vi "Robot Global Data.vi"() -> ()   [LabVIEW 2014]
doc: "This global VI can contain as many global variables as you need. Place a control on the panel, give it a good name. To read or write to it from a VI, drag the icon to the diagram of that VI. You can also drag from the project. Click on the node to change which global you access. You shouldn't have multiple locations writing to a global or it will cause a race-condition."
uses:
  <vilib>/Rock Robotics/WPI/DriverStation/WPI_DriverStationRobotMode2.ctl
  <vilib>/Rock Robotics/WPI/Camera/WPI_CameraImageSize.ctl
panel:
  out "Angle Kill":bool
  out "Chute Load Command":bool
  out "Gyro Angle":dbl
  out "Offset Pivot":bool
  out "Wheel Lock":bool
  in  "image size":T1=enum."320x240"
  out "Enable Vision":bool
  out "Zero Angle Target and Gyro":bool
  out "Manual Mode":bool
  out "Manual Elevator":dbl
  out "Rachet Up Position":dbl=750.0
  out "Feeder Mode":bool
  out "Tote Load Command":bool
  out "Elevator Kill Button":bool
  out "Wheel speed":dbl=1.0
  out "Wheels out":bool
  out "Wheels in":bool
  out "Spin Joy X":dbl
  out "Elevator PID Gains":T2={"proportional gain (Kc)"=1.0, "integral time (Ti, min)"=0.01, "derivative time (Td, min)"=0.0} {"derivative time (Td, min)" format="%.3f"; "integral time (Ti, min)" format="%.3f"; "proportional gain (Kc)" format="%.3f"}
  out "Turn PID Gains":T2={"proportional gain (Kc)"=1.0, "integral time (Ti, min)"=0.01, "derivative time (Td, min)"=0.0} {"derivative time (Td, min)" format="%.3f"; "integral time (Ti, min)" format="%.3f"; "proportional gain (Kc)" format="%.3f"}
  out "Base PID Gains":T2={"proportional gain (Kc)"=1.0, "integral time (Ti, min)"=0.01, "derivative time (Td, min)"=0.0} {"derivative time (Td, min)" format="%.3f"; "integral time (Ti, min)" format="%.3f"; "proportional gain (Kc)" format="%.3f"}
  out "Elevator Setpoint":dbl
  out "Rotation Correction Factor":dbl
  out "Closed Loop":bool=TRUE
  out "Robot Max Rate":dbl=200.0
  out "Record Data":bool
  out "Robot Timebase (ms)":u32=20
  out "Robot X Setpoint":dbl
  out "Robot Y Setpoint":dbl
  out "Angular Target":dbl
  in  "Robot Mode":T3
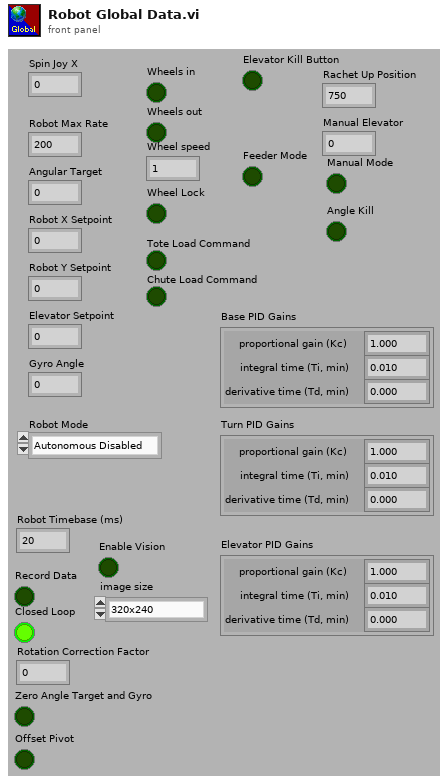
[diagram p1: front panel]
types:
  T1 = typedef "WPI_CameraImageSize.ctl" = enum16{"640x480", "320x240", "160x120", "Custom"}
  T2 = cluster{"proportional gain (Kc)":dbl, "integral time (Ti, min)":dbl, "derivative time (Td, min)":dbl}
  T3 = typedef "WPI_DriverStationRobotMode2.ctl" = enum16{"Autonomous Disabled", "Autonomous Enabled", "Teleop Disabled", "Teleop Enabled", "Disconnected", "Finish", "Test Disabled", "Test Enabled", "Emergency Stopped"}
diagram:
